vi "I2C Read.vi"(5 "Timeout (1000 ms)":u16=1000, 7 "I2C Channel":u8, 8 "Error In":errorcluster, 9 "Bytes To Read":u8, 10 "I2C Slave Address (0)":u8, 11 "LINX Resource":T1) -> (0 "Error Out":errorcluster, 2 "Data":u8[](array[numeric]), 3 "LINX Resource":T1)   [LabVIEW 2013, in "LVH-LINX.lvlib"]
doc: "Read the specified number of bytes from the I2C slave on the specified channel."
uses:
  <vilib>/LabVIEW Hacker/LINX/LVH-LINX.lvlib
  <vilib>/LabVIEW Hacker/LINX/Private/Type Defs/LINX Ref.ctl
  <vilib>/LabVIEW Hacker/LINX/Private/Type Defs/Platform.ctl
  <vilib>/LabVIEW Hacker/LINX/Private/Type Defs/Interface.ctl
  <vilib>/LabVIEW Hacker/LINX/Private/Device/Type Defs/LINX Device Config.ctl
  <vilib>/LabVIEW Hacker/LINX/Private/Device/Type Defs/TCP Config.ctl
  <vilib>/LabVIEW Hacker/LINX/Private/Type Defs/Device Family.ctl
  <vilib>/LabVIEW Hacker/LINX/Private/Type Defs/Peripheral.ctl
  <vilib>/LabVIEW Hacker/LINX/Private/Type Defs/Channel FGV States.ctl
  <vilib>/myRIO/Instrument Drivers/Onboard IO/I2C/typedefs/I2C Transfer Rate.ctl
  <vilib>/myRIO/Instrument Drivers/Onboard IO/I2C/typedefs/I2C Configuration.ctl
  <vilib>/myRIO/Common/Instrument Driver Framework/myRIO v1.0/I2C/typedefs/I2C Channels Enum.ctl
  <vilib>/myRIO/Common/Instrument Driver Framework/Utilities/typedefs/Generic FPGA Reference.ctl
  <vilib>/myRIO/Common/Instrument Driver Framework/Utilities/typedefs/myRIO v1.0 Reference.ctl
  <vilib>/myRIO/Common/Instrument Driver Framework/Utilities/typedefs/Hardware Version Enum.ctl
  <vilib>/myRIO/Common/Instrument Driver Framework/Utilities/typedefs/myRIO Generic Hardware Reference.ctl
  <vilib>/myRIO/Instrument Drivers/Onboard IO/I2C/typedefs/I2C Reference.ctl
  <vilib>/LabVIEW Hacker/LINX/Private/Device/Device.lvlib
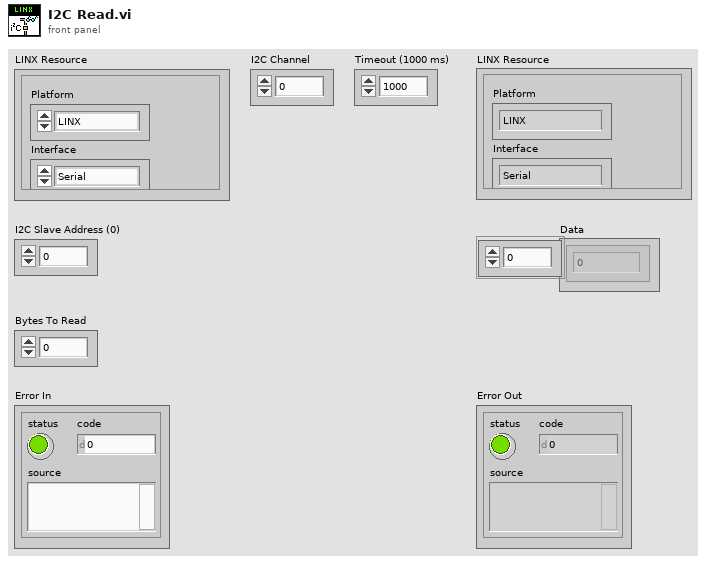
[diagram p1: front panel]
types:
  T1 = typedef "LVH-LINX.lvlib/LINX Ref.ctl" = cluster{"Platform":T2, "Interface":T3, "LINX Device Config":T4}
  T2 = typedef "LVH-LINX.lvlib/Platform.ctl" = enum16{"LINX", "myRIO"}
  T3 = typedef "LVH-LINX.lvlib/Interface.ctl" = enum16{"Serial", "TCP"}
  T4 = typedef "LVH-LINX.lvlib/Device.lvlib/LINX Device Config.ctl" = cluster{"Interface":T3, "COM Port":refnum<visa-resource-name>, "TCP Configuration":T5, "Device Family":T6, "Device ID":u8, "Device Name":string, "TCP Ref":refnum<k5>}
  T5 = typedef "LVH-LINX.lvlib/Device.lvlib/TCP Config.ctl" = cluster{"IP Address":string, "Port":u16}
  T6 = typedef "LVH-LINX.lvlib/Device Family.ctl" = enum8{"National Instruments", "Digilent", "Arduino"}
  T7 = typedef "LVH-LINX.lvlib/Peripheral.ctl" = enum8{"DI", "DO", "AI", "AO", "PWM", "QE", "UART", "I2C", "SPI", "CAN"}
  T8 = typedef "LVH-LINX.lvlib/Channel FGV States.ctl" = enum16{"Initialize", "Get", "Set"}
  T9 = typedef "I2C.lvlib/I2C Reference.ctl" = cluster{"myRIO Reference":T10, "I2C Channels Enum":T14, "I2C Configuration":T15}
  T10 = typedef "myRIO Generic Hardware Reference.ctl" = cluster{"myRIO Model":T11, "myRIO Hardware Reference":T12}
  T11 = typedef "Hardware Version Enum.ctl" = enum16{"Unknown", "myRIO-1900", "myRIO-1950"}
  T12 = typedef "myRIO v1.0 Reference.ctl" = cluster{"Generic FPGA Reference":T13, "Allow multiple opens":bool}
  T13 = typedef "Generic FPGA Reference.ctl" = refnum<k20>
  T14 = typedef "I2C Channels Enum.ctl" = enum16{"Not Connected", "A/I2C", "B/I2C"}
  T15 = typedef "I2C.lvlib/I2C Configuration.ctl" = cluster{"I2C Transfer Rate":T16}
  T16 = typedef "I2C.lvlib/I2C Transfer Rate.ctl" = enum16{"Standard Mode (100 kbps)", "Fast Mode (400 kbps)"}
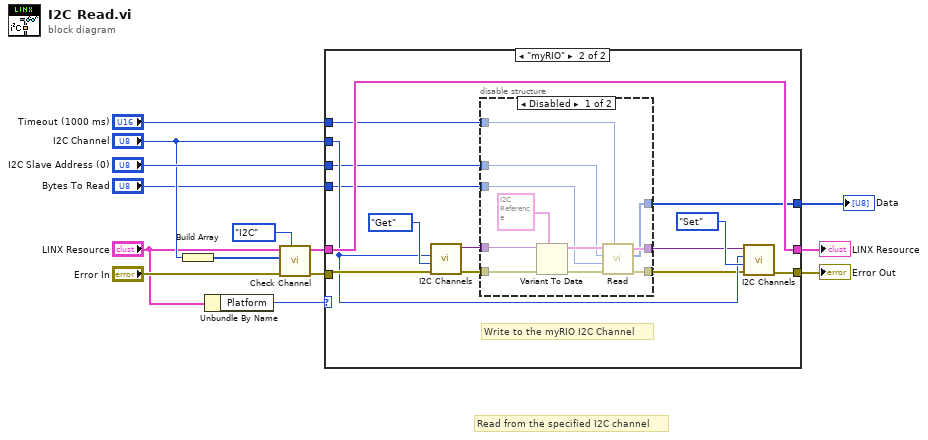
[diagram p0: block diagram]
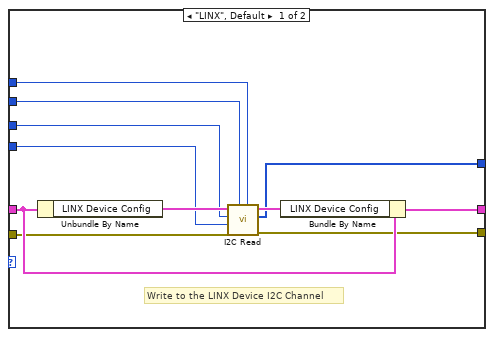
[diagram p2: hidden frame]
diagram:
  # "Read from the specified I2C channel"
  n1 = Build Array("I2C Channel") -> (w6:u8[])
  n2 = Unbundle By Name("LINX Resource") -> ("Platform"=w14:T2)
  n3 = call <vilib>:"Check Channel.vi"("Peripheral"=Peripheral."I2C", "Error In"="Error In", "Channels"=w6, "LINX Resource"="LINX Resource") -> ("Error Out"=w8:errorcluster, "LINX Resource"=w4:T1)  [unwired: 5 in, 1 out]
  n4 = case shown="\"myRIO\"" w14 {
    tunnel: w8 -> [w21 w35]
    tunnel: w4 -> [w25 w39]
    tunnel: [w20 w38] -> w13
    tunnel: [w24 w39] -> w12
    tunnel: "I2C Channel" -> [w19 w34]
    tunnel: "I2C Slave Address (0)" -> [w18 w31]
    tunnel: "Bytes To Read" -> [w17 w27]
    tunnel: "Timeout (1000 ms)" -> [w16 w28]
    tunnel: [w15 w26] -> w1
    frame "LINX", Default {
      # "Write to the LINX Device I2C Channel"
      n5 = Unbundle By Name(w25) -> ("LINX Device Config"=w23:T4)
      n6 = call <vilib>:"I2C Read.vi"("Timeout (1000 ms)"=w16, "I2C Channel (0)"=w19, "Error In"=w21, "Bytes To Read"=w17, "I2C Slave Address"=w18, "LINX Device Config"=w23) -> ("Error Out"=w20:errorcluster, "Data"=w15:u8[], "LINX Device Config"=w22:T4)  [unwired: 3 in]
      n7 = Bundle By Name(cluster=w25, "LINX Device Config"=w22) -> (w24:T1)
    }
    frame "myRIO" {
      # "Write to the myRIO I2C Channel"
      n8 = call <vilib>:"I2C Channels.vi"("Error In"=w35, "Channel State"=Channel_FGV_States."Get", "Channel Number"=w34) -> ("Error Out"=w33:errorcluster, "I2C Channel"=w32:variant)  [unwired: 7 in]
      n9 = disable-structure shown="Disabled" {
        disable-tunnel: w33 -> [w49 _]
        disable-tunnel: w32 -> [w48 _]
        disable-tunnel: w31 -> [w42 _]
        disable-tunnel: [w46 _] -> w30
        disable-tunnel: [w45 _] -> w29
        disable-tunnel: w28 -> [w44 _]
        disable-tunnel: w27 -> [w41 _]
        disable-tunnel: [w40 _] -> w26
        frame Disabled {
          n10 = Variant To Data(error in=w49, type=T9 {"myRIO Reference"={"myRIO Model"=enum."Unknown", "myRIO Hardware Reference"={"Generic FPGA Reference"=refnum, "Allow multiple opens"=FALSE}}, "I2C Channels Enum"=enum."Not Connected", "I2C Configuration"={"I2C Transfer Rate"=enum."Standard Mode (100 kbps)"}}, Variant=w48) -> (data=w43:T9, error out=w47:errorcluster)
          n11 = call <vilib>:"Read.vi"("Timeout ms (1000)"=w44, "error in (no error)"=w47, "Byte Count"=w41, "Slave Address (7-bit)"=w42, "I2C Ref In"=w43) -> ("error out"=w45:errorcluster, "Bytes Read"=w40:u8[], "I2C Ref Out"=w46:T9)  [unwired: 3 in]
        }
        frame Enabled {
        }
      }
      n12 = call <vilib>:"I2C Channels.vi"("Error In"=w29, "Channel State"=Channel_FGV_States."Set", "Channel Number"=w34, "I2C Channel"=w30) -> ("Error Out"=w38:errorcluster)  [unwired: 6 in, 1 out]
    }
  }
  "Error Out" <- w13
  "LINX Resource" <- w12
  "Data" <- w1
